vi "EOF Filter.vi"(3 "error in (no error)":errorcluster) -> (0 "error out":errorcluster, 1 "End-of-File?":bool)   [LabVIEW 2013]
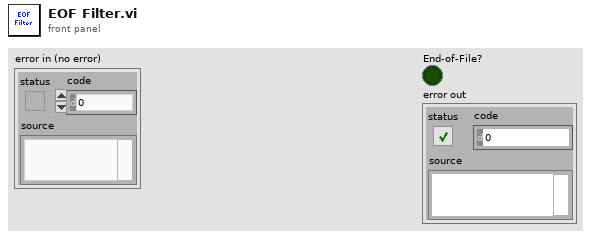
[diagram p1: front panel]
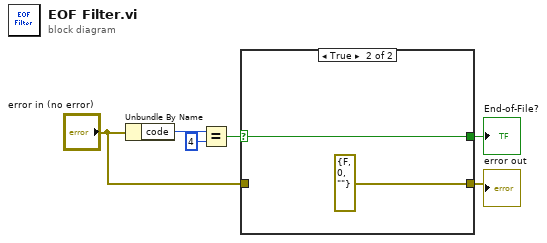
[diagram p0: block diagram]
diagram:
  n1 = Unbundle By Name("error in (no error)") -> ("code"=w6:i32)
  n2 = Equal?(x=w6, y=4) -> (x = y?=w4:bool)
  n3 = case shown="True" w4 {
    selector: w4 -> [w7 w9]
    tunnel: "error in (no error)" -> [w8 _]
    tunnel: [w8 errorcluster {"status"=FALSE, "code"=0, "source"=""} ("error constant")] -> w1
    tunnel: [w7 w9] -> w2
    frame False {
    }
    frame True {
    }
  }
  "End-of-File?" <- w2
  "error out" <- w1
